vi "upload.vi"(8 "error in (no error)":errorcluster, 11 "ICSettingsViewer in":refnum<class "ICSettingsViewer.lvclass">) -> (0 "error out":errorcluster, 3 "ICSettingsViewer out":refnum<class "ICSettingsViewer.lvclass">)   [LabVIEW 2009, in "Views.lvlib" / "Camera.lvlib" / "ICSettingsViewer.lvclass"]
uses:
  ICSettingsViewer.lvclass
  Tools/SettingsEventManager/SettingsEventsManager.lvclass
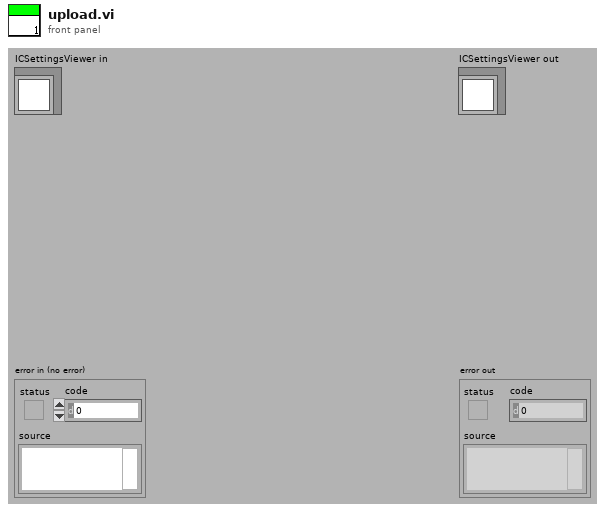
[diagram p1: front panel]
types:
  T1 = cluster{"settingsFrontEndEvents":cluster{"loadSettingsFromPath":refnum<user-event>, "lookUpElementEvent":refnum<user-event>, "saveSettings":refnum<user-event>, "loadSettings":refnum<user-event>, "close":refnum<user-event>, "replaceElement":refnum<user-event>, "findParentNodes":refnum<user-event>, "createNode":refnum<user-event>}, "settingBackEndEvents":cluster{"defaultSettingsPathRequest":refnum<user-event>, "searchResultEvent":refnum<user-event>, "settingsSaved":refnum<user-event>, "settingsLoaded":refnum<user-event>, "foundParentNode":refnum<user-event>}}
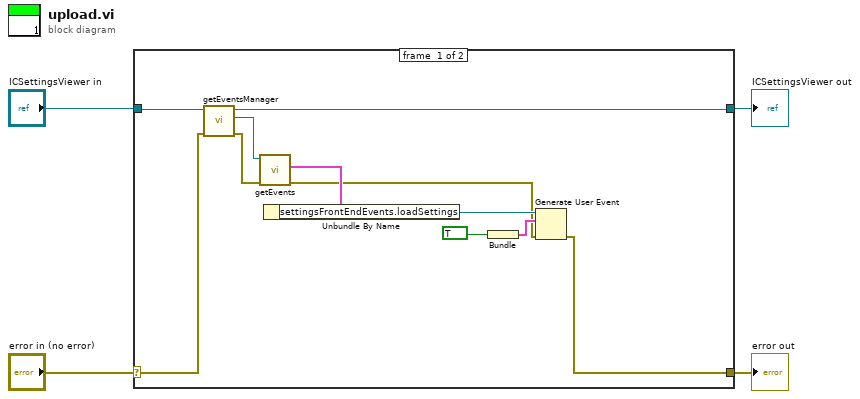
[diagram p0: block diagram]
diagram:
  n1 = case shown="No Error" "error in (no error)" {
    selector: "error in (no error)" -> [w11 w17]
    tunnel: [w5 w17] -> w3
    tunnel: [w12 w16] -> w1
    tunnel: "ICSettingsViewer in" -> [w13 w16]
    frame #0 {
      n2 = call-dynamic "getEventsManager.vi"("error in (no error)"=w11, "SettingsViewer.lvclass in"=w13) -> ("error out"=w14:errorcluster, "Tools.lvlib:Settings.lvlib:SettingsEventsManager.lvclass"=w15:refnum<class "SettingsEventsManager.lvclass">, "SettingsViewer.lvclass out"=w12:refnum<class "ICSettingsViewer.lvclass">)  [unwired: 7 in]
      n3 = call-dynamic "getEvents.vi"("error in (no error)"=w14, "SettingsEventsManager in"=w15) -> ("error out"=w6:errorcluster, "settingsEvents"=w10:T1)  [unwired: 7 in, 1 out]
      n4 = Unbundle By Name(w10) -> ("settingsFrontEndEvents.loadSettings"=w9:refnum<user-event>)
      n5 = Bundle(TRUE) -> (w7:cluster{bool})  [unwired: 1 in]
      n6 = Generate User Event(user event=w9, event data cluster=w7, error in=w6) -> (error out=w5:errorcluster)  [unwired: 1 out]
    }
    frame #1 {
    }
  }
  "error out" <- w3
  "ICSettingsViewer out" <- w1
